vi "Aero Cooling Valve Async.vi"() -> ()   [LabVIEW 2022 SP3]
uses:
  Aero Cooling Global.vi
panel:
  out "Dem Pos %":dbl
  out "Off Seconds":dbl format="%.1f"
  out "On seconds":dbl format="%.1f"
  in  "Min Valve Travel Time (s)":dbl=3.0
  in  "Total Cycle Time (s)":dbl=40.0
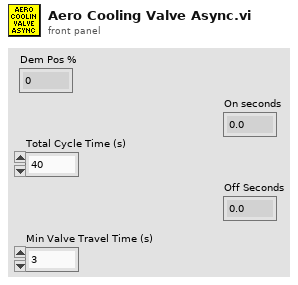
[diagram p1: front panel]
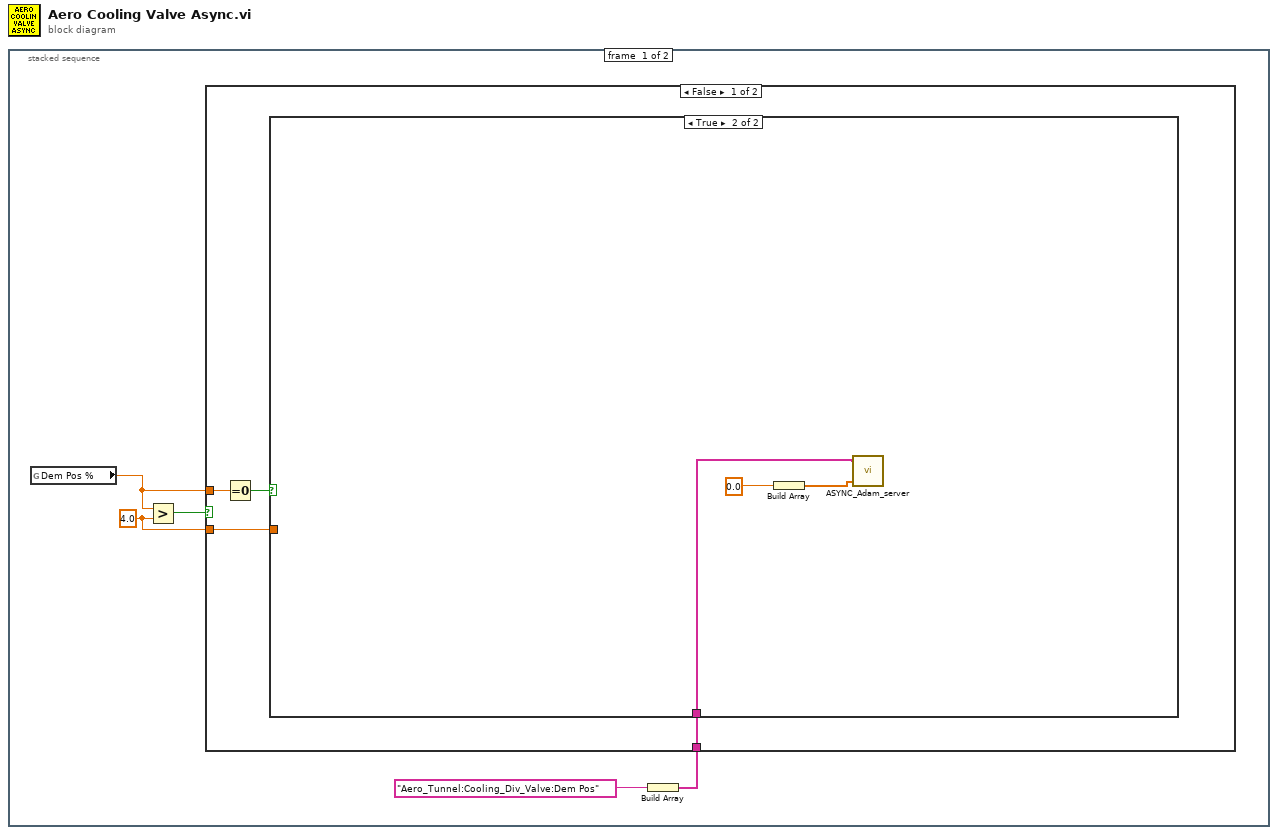
[diagram p0: block diagram]
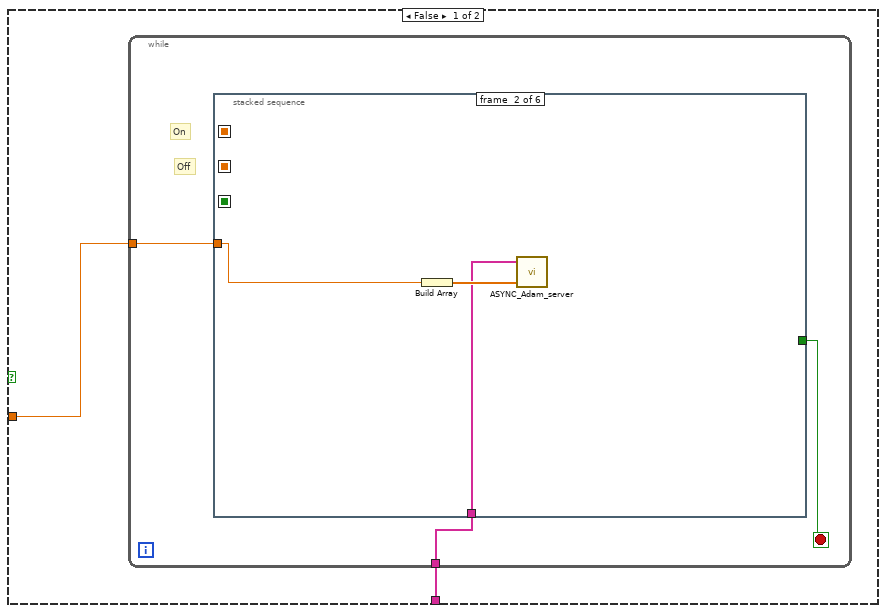
[diagram p2: hidden frame]
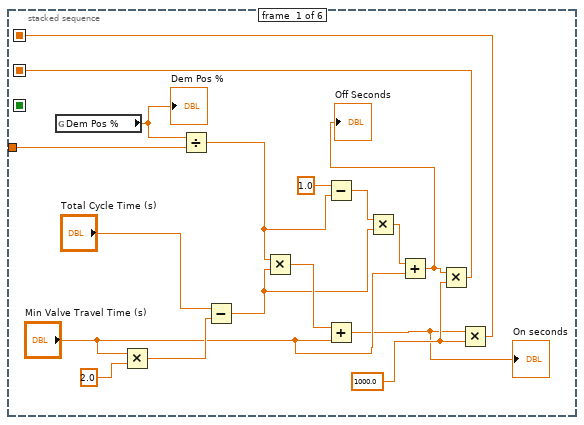
[diagram p3: hidden frame]
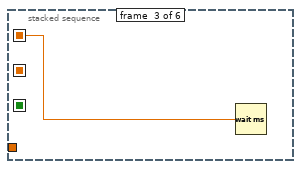
[diagram p4: hidden frame]
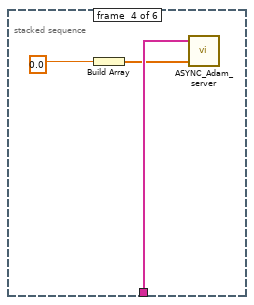
[diagram p5: hidden frame]
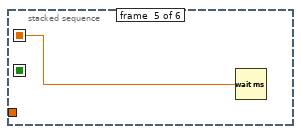
[diagram p6: hidden frame]
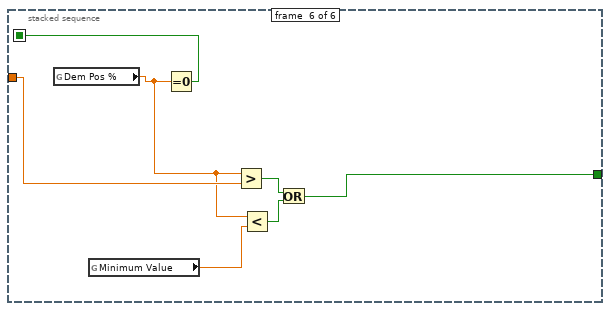
[diagram p7: hidden frame]
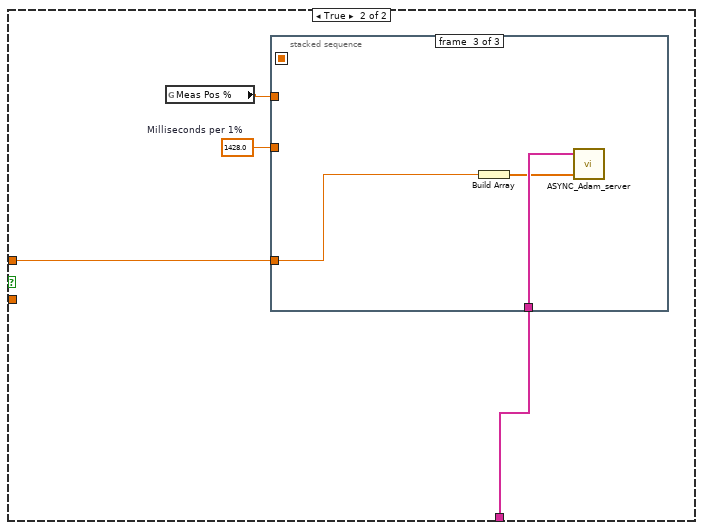
[diagram p8: hidden frame]
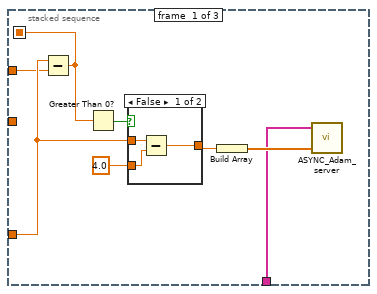
[diagram p9: hidden frame]
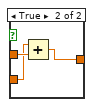
[diagram p10: hidden frame]
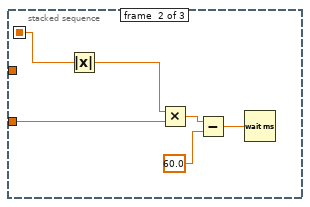
[diagram p11: hidden frame]
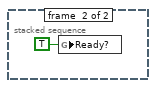
[diagram p12: hidden frame]
diagram:
  n1 = stacked-sequence {
    frame #0 {
      w1 = 4.0 ("y")
      n2 = global read "Aero Cooling Global.vi" "Dem Pos %"() -> (w3:dbl)
      n3 = Greater?(x=w3, y=w1) -> (0:w2:bool)
      n4 = Build Array("Aero_Tunnel:Cooling_Div_Valve:Dem Pos") -> (w4:string[])
      n5 = case shown="False" w2 {
        tunnel: w4 -> [w9 w53]
        tunnel: w3 -> [w6 w50]
        tunnel: w1 -> [w8 _]
        frame False {
          n6 = Equal To 0?(x=w6) -> (x = 0?=w7:bool)
          n7 = case shown="True" w7 {
            tunnel: w9 -> [w11 w48]
            tunnel: w8 -> [w10 _]
            frame False {
              n8 = while {
                tunnel: w11 -> [w14]
                tunnel: w10 -> [w12]
                stop <- w13 stop-if-true
                # "Off"
                # "On"
                n9 = stacked-sequence {
                  seq-local: [w25 _ _ _ _ _] -> [_ _ w35 _ _ _]
                  seq-local: [w17 _ _ _ _ _] -> [_ _ _ _ w39 _]
                  seq-local: [_ _ _ _ _ w40] -> [_ _ _ _ _ _]
                  tunnel: w14 -> [_ w33 _ w38 _ _]
                  tunnel: [_ _ _ _ _ w43] -> w13
                  tunnel: w12 -> [w27 w32 _ _ _ w46]
                  frame #0 {
                    w18 = 1000.0 ("y")
                    n10 = global read "Aero Cooling Global.vi" "Dem Pos %"() -> (w28:dbl)
                    "Dem Pos %" <- w28
                    n11 = Multiply(x="Min Valve Travel Time (s)", y=2.0) -> (x*y=w29:dbl)
                    n12 = Divide(x=w28, y=w27) -> (x/y=w23:dbl)
                    n13 = Subtract(x="Total Cycle Time (s)", y=w29) -> (x-y=w21:dbl)
                    n14 = Multiply(x=w23, y=w21) -> (x*y=w26:dbl)
                    n15 = Subtract(x=1.0, y=w23) -> (x-y=w22:dbl)
                    n16 = Add(x=w26, y="Min Valve Travel Time (s)") -> (x+y=w16:dbl)
                    "On seconds" <- w16
                    n17 = Multiply(x=w22, y=w21) -> (x*y=w20:dbl)
                    n18 = Add(x=w20, y="Min Valve Travel Time (s)") -> (x+y=w15:dbl)
                    "Off Seconds" <- w15
                    n19 = Multiply(x=w15, y=w18) -> (x*y=w17:dbl)
                    n20 = Multiply(x=w16, y=w18) -> (x*y=w25:dbl)
                  }
                  frame #1 {
                    n21 = Build Array(w32) -> (w34:dbl[])
                    n22 = call "ASYNC_Adam_server.vi"("Values"=w34, "Channel Names"=w33) -> ()  [unwired: 2 in, 2 out]
                  }
                  frame #2 {
                    n23 = Wait (ms)(milliseconds to wait=w35) -> ()  [unwired: 1 out]
                  }
                  frame #3 {
                    n24 = Build Array(0.0 ("y")) -> (w37:dbl[])
                    n25 = call "ASYNC_Adam_server.vi"("Values"=w37, "Channel Names"=w38) -> ()  [unwired: 2 in, 2 out]
                  }
                  frame #4 {
                    n26 = Wait (ms)(milliseconds to wait=w39) -> ()  [unwired: 1 out]
                  }
                  frame #5 {
                    n27 = global read "Aero Cooling Global.vi" "Dem Pos %"() -> (w41:dbl)
                    n28 = global read "Aero Cooling Global.vi" "Minimum Value"() -> (w42:dbl)
                    n29 = Equal To 0?(x=w41) -> (x = 0?=w40:bool)
                    n30 = Greater?(x=w41, y=w46) -> (0:w44:bool)
                    n31 = Less?(x=w41, y=w42) -> (x < y?=w45:bool)
                    n32 = Or(x=w44, y=w45) -> (x .or. y?=w43:bool)
                  }
                }
              }
            }
            frame True {
              n33 = Build Array(0.0 ("y")) -> (w47:dbl[])
              n34 = call "ASYNC_Adam_server.vi"("Values"=w47, "Channel Names"=w48) -> ()  [unwired: 2 in, 2 out]
            }
          }
        }
        frame True {
          w52 = 1428.0  # Milliseconds per 1%
          n35 = global read "Aero Cooling Global.vi" "Meas Pos %"() -> (w51:dbl)
          n36 = stacked-sequence {
            seq-local: [w54 _ _] -> [_ w69 _]
            tunnel: w53 -> [w57 _ w76]
            tunnel: w50 -> [w56 _ w74]
            tunnel: w52 -> [_ w70 _]
            tunnel: w51 -> [w55 _ _]
            frame #0 {
              n37 = Subtract(x=w56, y=w55) -> (x-y=w54:dbl)
              n38 = Greater Than 0?(x=w54) -> (x > 0?=w60:bool)
              n39 = case shown="False" w60 {
                tunnel: w56 -> [w64 w67]
                tunnel: 4.0 ("x") -> [w63 w66]
                tunnel: [w62 w65] -> w59
                frame False {
                  n40 = Subtract(x=w64, y=w63) -> (x-y=w62:dbl)
                }
                frame True {
                  n41 = Add(x=w66, y=w67) -> (x+y=w65:dbl)
                }
              }
              n42 = Build Array(w59) -> (w58:dbl[])
              n43 = call "ASYNC_Adam_server.vi"("Values"=w58, "Channel Names"=w57) -> ()  [unwired: 2 in, 2 out]
            }
            frame #1 {
              n44 = Absolute Value(x=w69) -> (abs(x)=w68:dbl)
              n45 = Multiply(x=w68, y=w70) -> (x*y=w72:dbl)
              n46 = Subtract(x=w72, y=60.0) -> (x-y=w73:dbl)
              n47 = Wait (ms)(milliseconds to wait=w73) -> ()  [unwired: 1 out]
            }
            frame #2 {
              n48 = Build Array(w74) -> (w75:dbl[])
              n49 = call "ASYNC_Adam_server.vi"("Values"=w75, "Channel Names"=w76) -> ()  [unwired: 2 in, 2 out]
            }
          }
        }
      }
    }
    frame #1 {
      n50 = global write "Aero Cooling Global.vi" "Ready?"(TRUE ("Ready?")) -> ()
    }
  }
